vi "Delay Loop seconds SubVi.vi"(1 "Loop Seconds Delay":i32=2000) -> ()   [LabVIEW 2013]
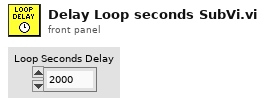
[diagram p1: front panel]
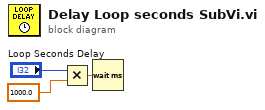
[diagram p0: block diagram]
diagram:
  n1 = Multiply(x="Loop Seconds Delay", y=1000.0) -> (x*y=w3:dbl)
  n2 = Wait (ms)(milliseconds to wait=w3) -> ()  [unwired: 1 out]
